vi "Spherical to Cartesian.vi"(4 "Spherical\nCoordinates":cluster{"rho":dbl, "theta":dbl, "phi":dbl}) -> (1 "Cartesian\nCoordinates":cluster{"x":dbl, "y":dbl, "z":dbl})   [LabVIEW 2013]
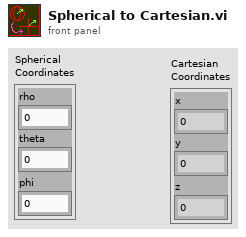
[diagram p1: front panel]
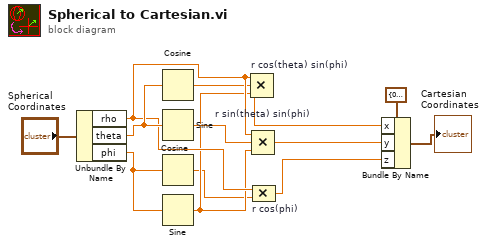
[diagram p0: block diagram]
diagram:
  n1 = Unbundle By Name("Spherical\nCoordinates") -> ("rho"=w6:dbl, "theta"=w8:dbl, "phi"=w7:dbl)
  n2 = Cosine(x=w8) -> (cos(x)=w4:dbl)
  n3 = Sine(x=w8) -> (sin(x)=w3:dbl)
  n4 = Cosine(x=w7) -> (cos(x)=w1:dbl)
  n5 = Sine(x=w7) -> (sin(x)=w2:dbl)
  n6 = Compound Arithmetic op=MULTIPLY "r cos(theta) sin(phi)"(w6, w4, w2) -> (w11:dbl)
  n7 = Compound Arithmetic op=MULTIPLY "r sin(theta) sin(phi)"(w6, w3, w2) -> (w10:dbl)
  n8 = Compound Arithmetic op=MULTIPLY "r cos(phi)"(w6, w1) -> (w5:dbl)
  n9 = Bundle By Name(cluster=cluster{"x":dbl, "y":dbl, "z":dbl} {"x"=0.0, "y"=0.0, "z"=0.0} ("input cluster"), "x"=w11, "y"=w10, "z"=w5) -> (→"Cartesian\nCoordinates":cluster{"x":dbl, "y":dbl, "z":dbl})
